vi "Stop Core.vi"(10 "final error code":i32, 11 "Log in":refnum<class "Log.lvclass">) -> (3 "Log out":refnum<class "Log.lvclass">)   [LabVIEW 2020, in "Log.lvlib" / "Log.lvclass"]
doc: "(<B>Filename</B>: Actor Framework.lvlib:Actor.lvclass:Stop Core.vi)\n\nDefines what the actor does before it stops. Use the <B>final error code</B> input to determine whether the actor shut down in response to an error.\n\nBy default, this method passes the Stop message along to all auto-stop nested actors. A descendant class may override this method to define additional behavior, such as shutting down any processes the actor initiated in its override of the Actor Core method."
uses:
  Log.lvclass
  <vilib>/ActorFramework/Actor/Actor.lvclass
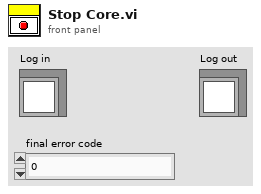
[diagram p1: front panel]
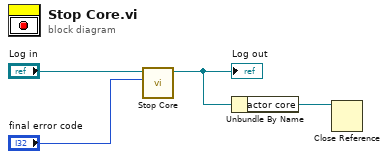
[diagram p0: block diagram]
diagram:
  n1 = call-parent "Stop Core.vi"("final error code"="final error code", "Actor in"="Log in") -> ("Actor out"=w1:refnum<class "Log.lvclass">)  [unwired: 9 in]
  "Log out" <- w1
  n2 = Unbundle By Name(w1) -> ("actor core"=w2:refnum<vi>)
  n3 = Close Reference(reference=w2) -> ()  [unwired: 1 in, 1 out]
